vi "状态机.vi"   [LabVIEW 2018]
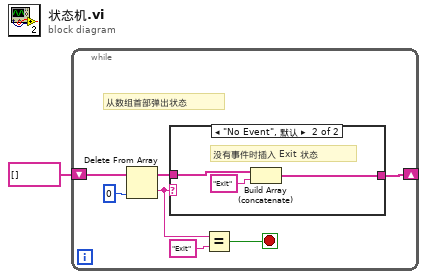
[diagram p0: block diagram]
diagram:
  n1 = while {
    shift-right: [w6] -> _
    shift-left: string[] [] -> [w8]
    stop <- w2 stop-if-true
    # "从数组首部弹出状态"
    n2 = Delete From Array(array=w8, index=0 ("索引")) -> (deleted portion=w4:string, array with subset deleted=w5:string[])  [unwired: 1 in]
    n3 = case shown="\"No Event\", 默认" w4 {
      tunnel: [_ w10] -> w6
      tunnel: w5 -> [_ w9]
      frame "假" {
      }
      frame "No Event", Default {
        # "没有事件时插入 Exit 状态"
        n4 = Build Array (concatenate)(w9, "Exit" ("元素")) -> (w10:string[])
      }
    }
    n5 = Equal?(x=w4, y="Exit") -> (x = y?=w2:bool)
  }
